vi "Set Bias Voltage.vi"(8 "error in (no error)":errorcluster, 9 "Channel":i32, 10 "Bias Voltage (V)":dbl, 11 "VoltageUpdate in":refnum<class "VoltageUpdate.lvclass">) -> (0 "error out":errorcluster, 3 "VoltageUpdate out":refnum<class "VoltageUpdate.lvclass">)   [LabVIEW 2016, in "VoltageUpdate.lvclass"]
uses:
  VoltageUpdate.lvclass
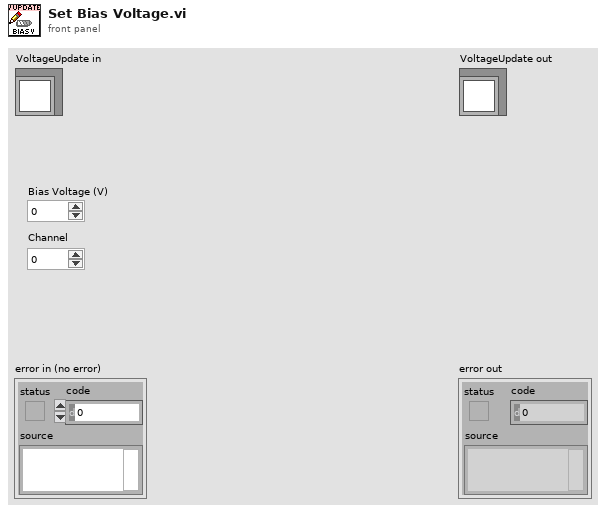
[diagram p1: front panel]
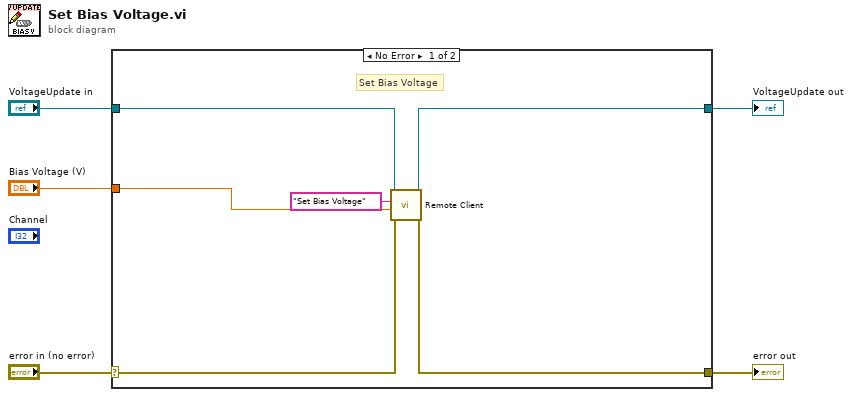
[diagram p0: block diagram]
diagram:
  n1 = case shown="No Error" "error in (no error)" {
    selector: "error in (no error)" -> [w7 w13]
    tunnel: [w6 w13] -> w4
    tunnel: [w8 w12] -> w3
    tunnel: "VoltageUpdate in" -> [w9 w12]
    tunnel: "Bias Voltage (V)" -> [w11 _]
    frame No Error {
      # "Set Bias Voltage"
      n2 = call-dynamic "Remote Client.vi"("error in (no error)"=w7, "Data"=w11, "Command"="Set Bias Voltage", "Instrument in"=w9) -> ("error out"=w6:errorcluster, "Instrument out"=w8:refnum<class "VoltageUpdate.lvclass">)  [unwired: 4 in, 2 out]
    }
    frame Error {
    }
  }
  "error out" <- w4
  "VoltageUpdate out" <- w3
